vi "1B_AnalyzeAmplitudeRamp_CalcTimeOffset.vi"(0 "Ramp Duration ( sec )":dbl=10.0, 1 "Offset Calculation Method":T3=enum."Precise", 2 "Resampling \nStrength":T2=enum."4", 3 "Smoothing Strength":T1=enum."50", 5 "DAQ":waveform(dbl)[](array[waveform])=[{"t0"=timestamp(3464860426.1720004 s since 1904-01-01), "dt"=3.8400000000000005e-06, "Y"=array[16000 elements]}, {"t0"=timestamp(3464860427.2660003 s since 1904-01-01), "dt"=3.8400000000000005e-06, "Y"=array[16000 elements]}, {"t0"=timestamp(3464860428.3440003 s since 1904-01-01), "dt"=3.8400000000000005e-06, "Y"=array[16000 elements]}, {"t0"=timestamp(3464860429.453 s since 1904-01-01), "dt"=3.8400000000000005e-06, "Y"=array[16000 elements]}, {"t0"=timestamp(3464860430.563 s since 1904-01-01), "dt"=3.8400000000000005e-06, "Y"=array[16000 elements]}, {"t0"=timestamp(3464860431.6720004 s since 1904-01-01), "dt"=3.8400000000000005e-06, "Y"=array[16000 elements]}, {"t0"=timestamp(3464860432.766 s since 1904-01-01), "dt"=3.8400000000000005e-06, "Y"=array[16000 elements]}, {"t0"=timestamp(3464860433.8750005 s since 1904-01-01), "dt"=3.8400000000000005e-06, "Y"=array[16000 elements]}, {"t0"=timestamp(3464860434.9690003 s since 1904-01-01), "dt"=3.8400000000000005e-06, "Y"=array[16000 elements]}], 7 "Input \nWaveform \nRepetitions":i32=4, 9 "Ramp End Pulse Characteristics":T4={"Pulses per Cycle"=4, "Load Resistance (Ohms)"=750.0, "Krec Value"=2, "Recovery Mode (T=Active)"=TRUE, "Amps"=[0.01, 0.008, 0.005, 0.002]} {"Amps" format="%#_6p"}) -> (8 "Best Measurement Time Offset ( sec )":dbl=1.2 format="%#.3p")   [LabVIEW 2010]
uses:
  1B_Offset Calculation Method.ctl
  1B_Resample Strength.ctl
  FilterStrength.ctl
panel:
  out "Measurement Offset Times ( sec )":dbl[](array[numeric])
  out "error [ A ]":dbl[](array[numeric]) format="%#.3p"
  # "Enter Target Current\nfor each in array below"
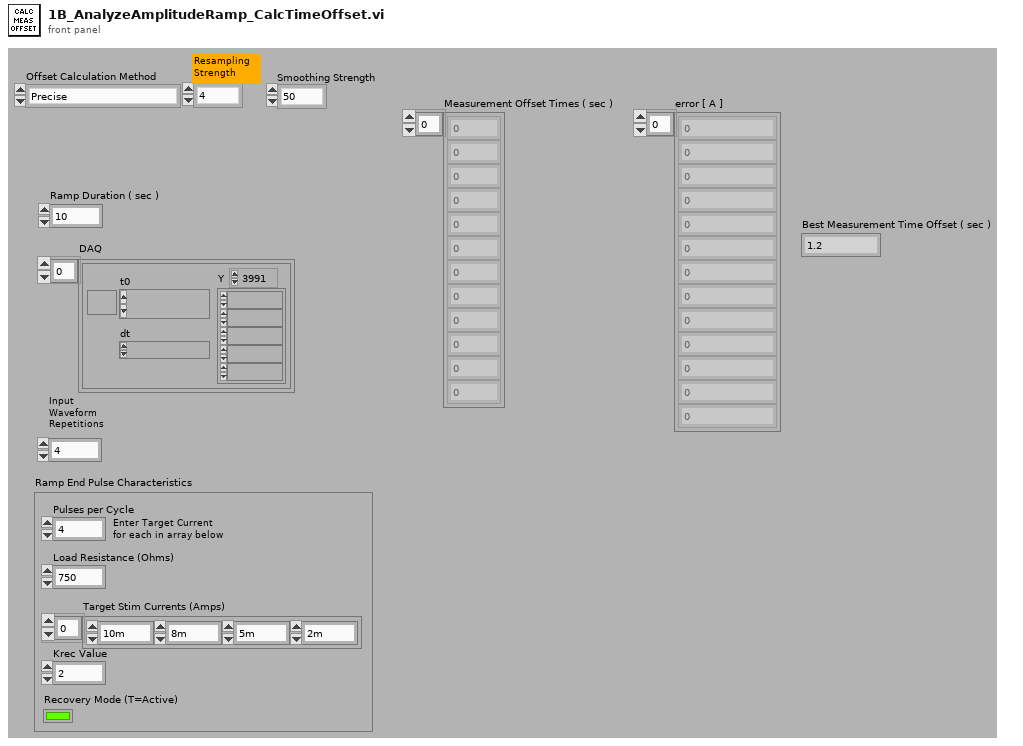
[diagram p1: front panel]
types:
  T1 = typedef "FilterStrength.ctl" = enum16{"Off", "10", "20", "50", "100", "200", "500", "1000"}
  T2 = typedef "1B_Resample Strength.ctl" = enum16{"Off", "2", "4", "8", "16", "32"}
  T3 = typedef "1B_Offset Calculation Method.ctl" = enum16{"Obsolete", "Precise", "Simple"}
  T4 = cluster{"Pulses per Cycle":i32, "Load Resistance (Ohms)":dbl, "Krec Value":i32, "Recovery Mode (T=Active)":bool, "Amps":dbl[]}
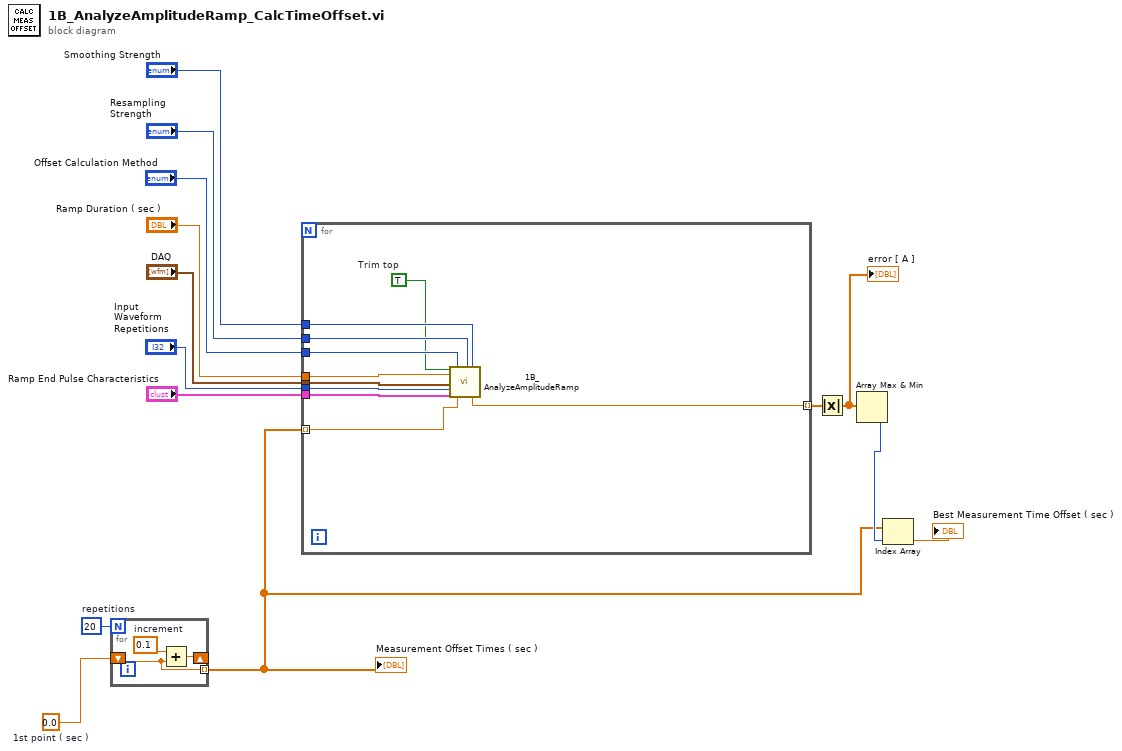
[diagram p0: block diagram]
diagram:
  w6 = 0.0  # 1st point ( sec )
  w7 = 20  # repetitions
  n1 = for {
    N: w7 -> [_]
    shift-right: [w15] -> _
    shift-left: w6 -> [w16]
    tunnel: [w16] -> w1 mode=indexing
    w17 = 0.1  # increment
    n2 = Add(x=w17, y=w16) -> (x+y=w15:dbl)
  }
  "Measurement Offset Times ( sec )" <- w1
  n3 = for {
    tunnel: "DAQ" -> [w27]
    tunnel: "Input \nWaveform \nRepetitions" -> [w26]
    tunnel: "Ramp Duration ( sec )" -> [w25]
    tunnel: "Ramp End Pulse Characteristics" -> [w24]
    tunnel: "Offset Calculation Method" -> [w23]
    tunnel: "Resampling \nStrength" -> [w22]
    tunnel: "Smoothing Strength" -> [w21]
    tunnel: w1 -> [w19] mode=indexing
    tunnel: [w20] -> w5 mode=indexing
    w18 = TRUE  # Trim top
    n4 = call "1B_AnalyzeAmplitudeRamp.vi"("Trim top"=w18, "Ramp Duration ( sec )"=w25, "DAQ"=w27, "Input \nWaveform \nRepetitions"=w26, "Ramp End Pulse Characteristics"=w24, "Offset Calculation Method"=w23, "Measurement Time Offset ( sec )"=w19, "Resampling \nStrength"=w22, "Smoothing Strength"=w21) -> ("P1 mean error [ A ]"=w20:dbl)  [unwired: 4 in, 6 out]
  }
  n5 = Absolute Value(x=w5) -> (abs(x)=w4:dbl[])
  "error [ A ]" <- w4
  n6 = Array Max & Min(array=w4) -> (min index (indices)=w3:i32)  [unwired: 3 out]
  n7 = Index Array(array=w1, index=w3) -> (element=→"Best Measurement Time Offset ( sec )":dbl)
